vi "combine_csv.vi"() -> ()   [LabVIEW 2019]
uses:
  <vilib>/Utility/file.llb/Write Delimited Spreadsheet (string).vi
panel:
  out "error out":errorcluster
  in  "Data folder (containing csv files)":path=path "C:/Users/Naomi Tan/Documents/Gillette/MH6/videos/Annotations/cropped_data"
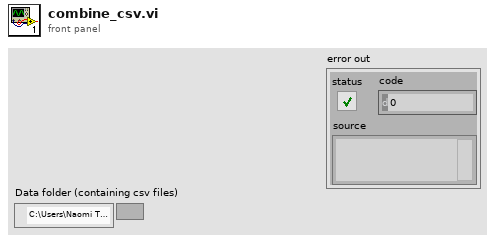
[diagram p1: front panel]
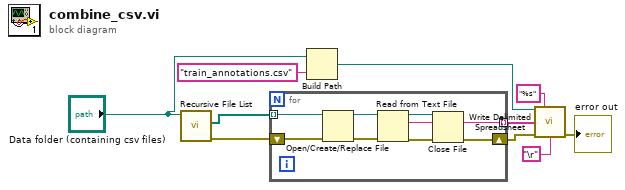
[diagram p0: block diagram]
diagram:
  n1 = call <vilib>:"Recursive File List.vi"("Folder Path"="Data folder (containing csv files)") -> ("error out"=w10:errorcluster, "All Files in Dir"=w9:path[])  [unwired: 6 in, 3 out]
  n2 = for {
    tunnel: w9 -> [w14] mode=indexing
    tunnel: [w18] -> w8 mode=indexing
    shift-right: [w11] -> w2
    shift-left: w10 -> [w15]
    n3 = Open/Create/Replace File(file path (use dialog)=w14, error in=w15) -> (refnum out=w17:refnum<file>, error out=w16:errorcluster)  [unwired: 4 in, 1 out]
    n4 = Read from Text File(file (use dialog)=w17, error in=w16) -> (refnum out=w13:refnum<file>, text=w18:string, error out=w12:errorcluster)  [unwired: 2 in, 1 out]
    n5 = Close File(refnum=w13, error in=w12) -> (error out=w11:errorcluster)  [unwired: 1 out]
  }
  n6 = Build Path(base path="Data folder (containing csv files)", name or relative path="train_annotations.csv") -> (appended path=w4:path)
  n7 = call-poly <vilib>:"Write Delimited Spreadsheet.vi"("file path (dialog if empty)"=w4, "format (%s)"="%s", "1D data"=w8, "error in (no error)"=w2, "delimiter (\\t)"="\r") -> ("error out"=→"error out":errorcluster)  [unwired: 9 in, 1 out]
